vi "Traffic Light Automatic Control - Cluster, ENUM & Case Structure.vi"() -> ()   [LabVIEW 2016]
panel:
  in  "stop":bool
  out "Signal":T1
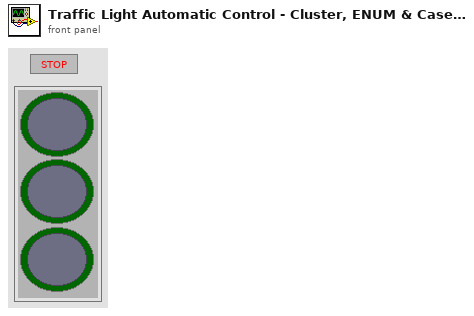
[diagram p1: front panel]
types:
  T1 = cluster{"Boolean":bool, "Boolean 2":bool, "Boolean 3":bool}
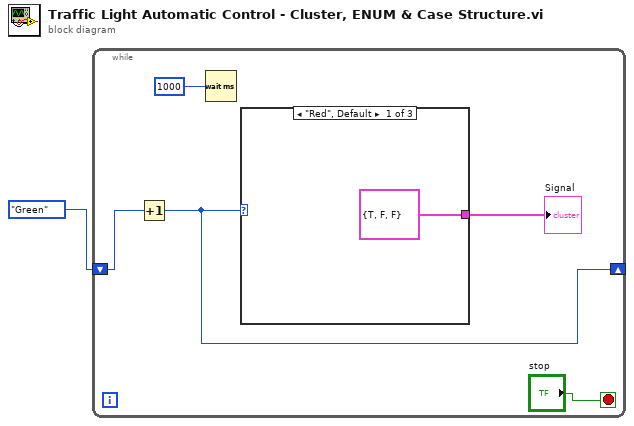
[diagram p0: block diagram]
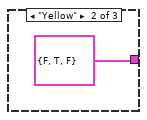
[diagram p2: hidden frame]
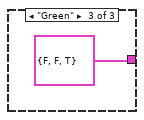
[diagram p3: hidden frame]
diagram:
  n1 = while {
    shift-right: [w5] -> _
    shift-left: enum16{"Red", "Yellow", "Green"}."Green" ("Enum") -> [w2]
    stop <- "stop" stop-if-true
    n2 = Increment(x=w2) -> (x+1=w5:enum16{"Red", "Yellow", "Green"})
    n3 = Wait (ms)(milliseconds to wait=1000) -> ()  [unwired: 1 out]
    n4 = case shown="\"Red\", Default" w5 {
      tunnel: [cluster{"Red":bool, "Yellow":bool, "Green":bool} {"Red"=TRUE, "Yellow"=FALSE, "Green"=FALSE} ("Signal 2") cluster{"Red":bool, "Yellow":bool, "Green":bool} {"Red"=FALSE, "Yellow"=TRUE, "Green"=FALSE} ("Signal 2") cluster{"Red":bool, "Yellow":bool, "Green":bool} {"Red"=FALSE, "Yellow"=FALSE, "Green"=TRUE} ("Signal 2")] -> w6
      frame "Red", Default {
      }
      frame "Yellow" {
      }
      frame "Green" {
      }
    }
    "Signal" <- w6
  }
